vi "get_as_SpaceVectors.vi"(8 "error in (no error)":errorcluster, 11 "TrajectoryDL091126GenericVoxel in":refnum<class "TrajectoryDL091126GenericVoxel.lvclass">) -> (0 "error out":errorcluster, 1 "number of voxels":i32, 2 "voxels":refnum<class "SpaceVector.lvclass">[](array[class]), 3 "TrajectoryDL091126GenericVoxel out":refnum<class "TrajectoryDL091126GenericVoxel.lvclass">)   [LabVIEW 2010, in "TrajectoryDL091126GenericVoxel.lvclass"]
uses:
  TrajectoryDL091126GenericVoxel.lvclass
  common/classes/SpaceVector/SpaceVector/SpaceVector.lvclass
  common/enumerations/functional_global_action_enum.ctl
  common/enumerations/x_y_z_enumeration.ctl
  common/classes/ErrorController/ErrorController/class_data.vi
  common/classes/ErrorController/ErrorController/ErrorController.lvclass
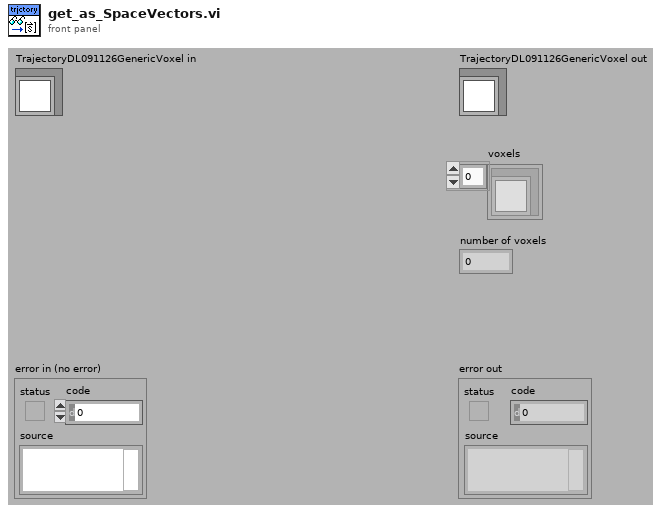
[diagram p1: front panel]
types:
  T1 = typedef "x_y_z_enumeration.ctl" = enum16{"x", "y", "z"}
  T2 = typedef "functional_global_action_enum.ctl" = enum16{"get", "set", "reset"}
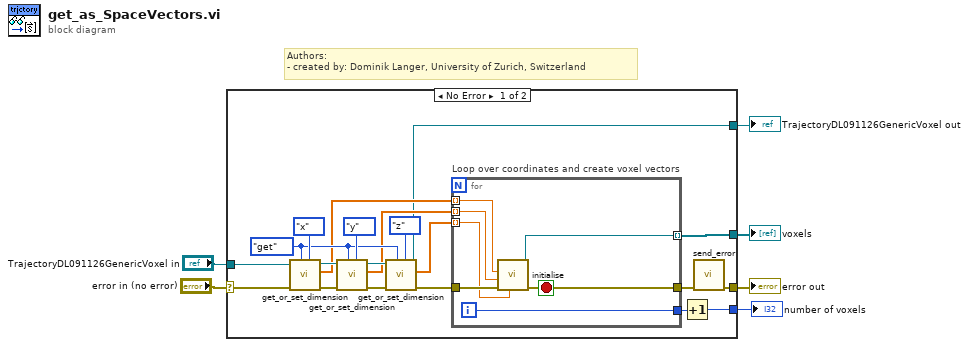
[diagram p0: block diagram]
diagram:
  # "Authors: \n- created by: Dominik Langer, University of Zurich, Switzerland"
  n1 = case shown="No Error" "error in (no error)" {
    selector: "error in (no error)" -> [w18 w35]
    tunnel: [w8 w35] -> w5
    tunnel: [w11 w34] -> w3
    tunnel: "TrajectoryDL091126GenericVoxel in" -> [w12 w34]
    tunnel: [w13 _] -> w2
    tunnel: [w9 _] -> w1
    frame No Error {
      w19 = functional_global_action_enum."get" ("action")
      n2 = call-dynamic "get_or_set_dimension.vi"("dimension"=x_y_z_enumeration."x", "action"=w19, "error in (no error)"=w18, "GenericTrajectory in"=w12) -> ("error out"=w26:errorcluster, "pixel values out (single dimension)"=w16:dbl[unit][], "GenericTrajectory out"=w24:refnum<class "TrajectoryDL091126GenericVoxel.lvclass">)  [unwired: 5 in]
      n3 = call-dynamic "get_or_set_dimension.vi"("dimension"=x_y_z_enumeration."y", "action"=w19, "error in (no error)"=w26, "GenericTrajectory in"=w24) -> ("error out"=w25:errorcluster, "pixel values out (single dimension)"=w15:dbl[unit][], "GenericTrajectory out"=w23:refnum<class "TrajectoryDL091126GenericVoxel.lvclass">)  [unwired: 5 in]
      n4 = call-dynamic "get_or_set_dimension.vi"("dimension"=x_y_z_enumeration."z", "action"=w19, "error in (no error)"=w25, "GenericTrajectory in"=w23) -> ("error out"=w17:errorcluster, "pixel values out (single dimension)"=w14:dbl[unit][], "GenericTrajectory out"=w11:refnum<class "TrajectoryDL091126GenericVoxel.lvclass">)  [unwired: 5 in]
      n5 = for "Loop over coordinates and create voxel vectors" {
        tunnel: w16 -> [w32] mode=indexing
        tunnel: w15 -> [w31] mode=indexing
        tunnel: w14 -> [w30] mode=indexing
        tunnel: [w29] -> w13 mode=indexing
        tunnel: [w28] -> w10
        tunnel: w17 -> [w33]
        tunnel: [w27] -> w7
        i -> [w28]
        stop <- w27 stop-if-true
        n6 = call "initialise.vi"("z"=w30, "error in (no error)"=w33, "y"=w31, "x"=w32) -> ("error out"=w27:errorcluster, "SpaceVector out"=w29:refnum<class "SpaceVector.lvclass">)  [unwired: 6 in]
      }
      n7 = Increment(x=w10) -> (x+1=w9:i32)
      n8 = call "send_error.vi"("error in (no error)"=w7) -> ("error out"=w8:errorcluster)  [unwired: 10 in]
    }
    frame Error {
    }
  }
  "error out" <- w5
  "TrajectoryDL091126GenericVoxel out" <- w3
  "voxels" <- w2
  "number of voxels" <- w1
